vi "Crio9067_12chan.vi"() -> ()   [LabVIEW 2014]
uses:
  <vilib>/rvi/eio/nirviErrorMerge/nirviErrorMerge.xnode
  <vilib>/rvi/eio/common/nirviEmuClasses.ctl
  <vilib>/rvi/eio/common/nirviEmuTemplateMethod_errors.vi
  <vilib>/rvi/eio/nirviEIOMethodImplementation/nirviEIOMethodImplementation.xnode
  <vilib>/eio/EIOGrowableMethodNode/genericMethod/EIOGrowableMethodNode.xnode
  <vilib>/rvi/DataTransferAndStorage/Container/XNode/niFpgaContainer.xnode
  <vilib>/eio/EIONode/EIONode.xnode
  <vilib>/rvi/interface/RandomDataEmulation/nirviRandomDataFpgaReadWriteTemplate.vi
panel:
  in  "User Fpga Led":bool
  out "Chassis Temperature":i16
  in  "System Reset":bool
  in  "Sample Period (uSec)":u32=2
  out "Timed Out":bool
  out "Overwrite":bool
  out "Sample Gated":bool
  in  "USER FPGA LED":bool
  in  "Boolean":bool
  out "Stopped":bool
  out "nChannels":i32=8
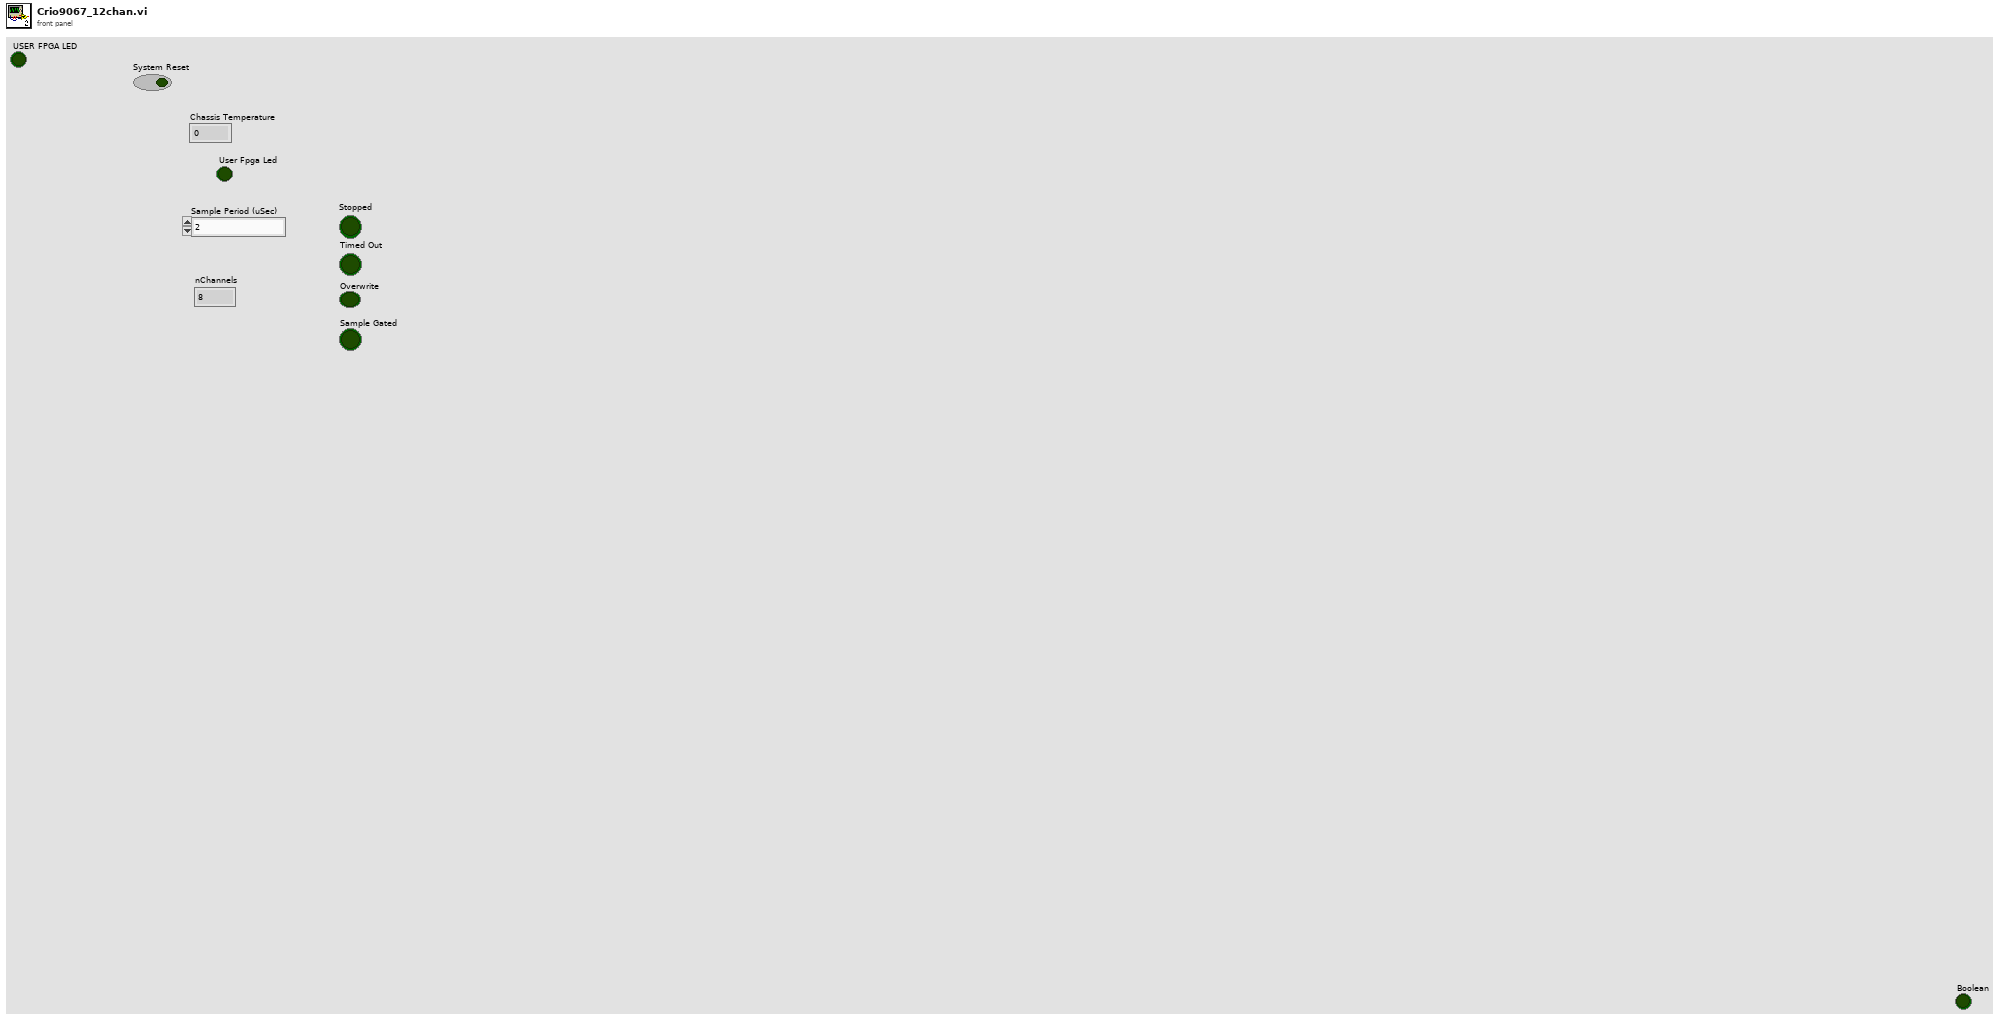
[diagram p1: front panel]
types:
  T1 = typedef "nirviEmuClasses.ctl" = enum16{"IO Read", "IO Write", "Method", "Property Read", "Property Write"}
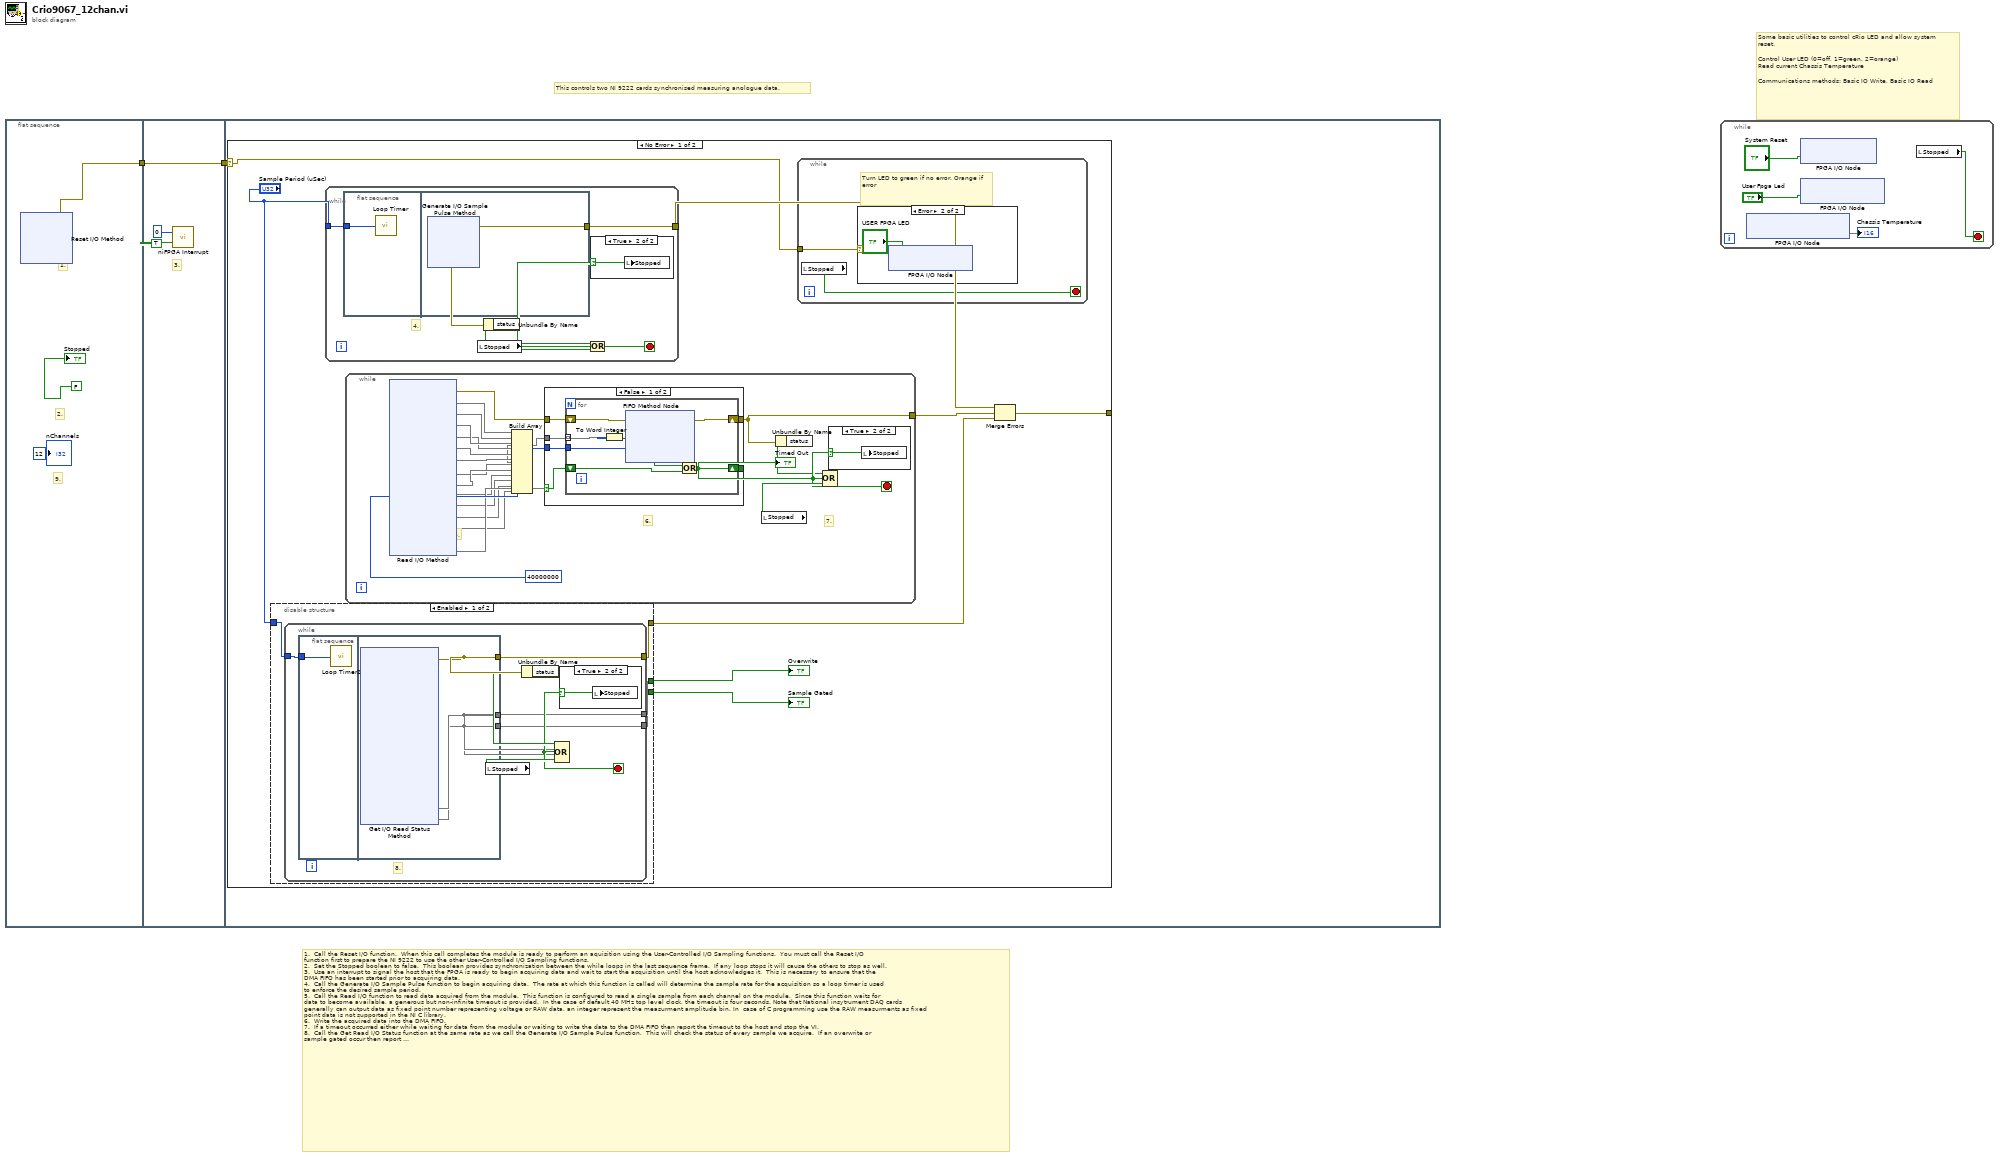
[diagram p0: block diagram]
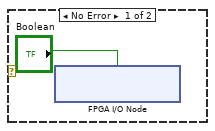
[diagram p2: hidden frame]
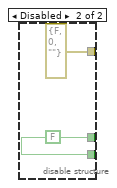
[diagram p4: hidden frame]
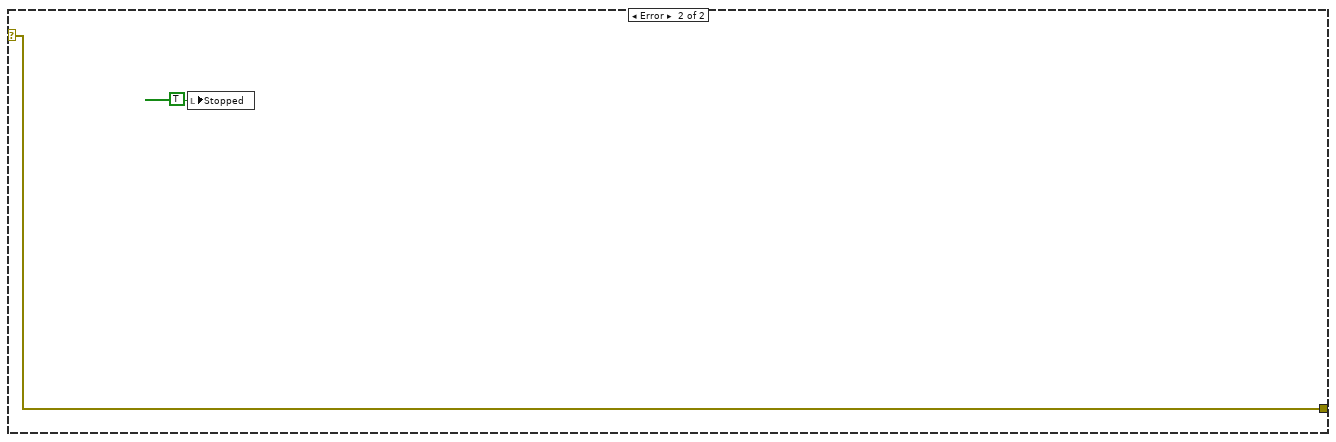
[diagram p8: hidden frame]
diagram:
  # "Some basic utilities to control cRio LED and allow system reset. \n\nControl User LED (0=off, 1=green, 2=orange)\nRead current Chassis Temperature\n\nCommunications methods: Basic IO Write, Basic IO Read"
  # "This controls two NI 9222 cards synchronised measuring anologue data."
  # "1.  Call the Reset I/O function.  When this call completes the module is ready to perform an aquisition using the User-Controlled I/O Sampling functions.  You must call the Reset I/O \nfunction first to prepare the NI 9222 to use the other User-Controlled I/O Sampling functions.\n2.  Set the Stopped boolean to false.  This boolean provides synchronization between the while loops in the last sequence frame.  If any loop stops it will cause the others to stop as well.\n3.  Use an interrupt to signal the host that the FPGA is ready to begin acquiring data and wait to start the acquisition until the host acknowledges it.  This is necessary to ensure that the \nDMA FIFO has been started prior to acquiring data.\n4.  Call the Generate I/O Sample Pulse function to begin acquiring data.  The rate at which this function is called will determine the sample rate for the acquisition so a loop timer is used\nto enforce the desired sample period.\n5.  Call the Read I/O function to read data acquired from the module.  This function is configured to read a single sample from each channel on the module.  Since this function waits for\ndata to become available, a generous but non-infinite timeout is provided.  In the case of default 40 MHz top level clock, the timeout is four seconds. Note that National insytrument DAQ cards \ngenerally can output data as fixed point number representing voltage or RAW data, an integer represent the measurment amplitude bin. In  case of C programming use the RAW measurments as fixed \npoint data is not supported in the NI C library. \n6.  Write the acquired data into the DMA FIFO.\n7.  If a timeout occurred either while waiting for data from the module or waiting to write the data to the DMA FIFO then report the timeout to the host and stop the VI.\n8.  Call the Get Read I/O Status function at the same rate as we call the Generate I/O Sample Pulse function.  This will check the status of every sample we acquire.  If an overwrite or \nsample gated occur then report the status to the host and stop the VI.  This loop is encased in a diagram disable struction to make it easily removable from the application.  Calling the \nGet Read I/O Status function is useful for development and debugging but not strictly necessary for deployment if there is no variable timing in the application.  In the above example, it\nis not possible to get a sample gated status unless the top loop's sample period is less than the minimum sample period supported by the module.  However, this application could \nproduce an overwrite status if the host VI cannot read from the DMA FIFO fast enough.\n9. I constant indicating the number of channels the FPGA is recording from. This is manually set."
  n1 = flat-sequence {
    tunnel: [w4] -> w2
    tunnel: w2 -> [w70]
    tunnel: [w70] -> w1
    tunnel: w1 -> [w73]
    frame #0 {
      # "9."
      # "2."
      # "1."
      n2 = xnode "Reset I/O Method"() -> ("error out"=w4:errorcluster)  [unwired: 1 in]
      "Stopped" <- FALSE ("Stopped")
      "nChannels" <- 12
    }
    frame #1 {
      # "3."
      n3 = call <vilib>:"niFPGA Interrupt.vi"("Wait Until Cleared (F)"=TRUE ("Wait Until Cleared"), "IRQ Number (0)"=u8 0 ("IRQ Number")) -> ()  [unwired: 1 in]
    }
    frame #2 {
      n4 = case shown="No Error" w73 {
        selector: w73 -> [w74 w1114]
        tunnel: [w78 w1114] -> _
        frame No Error {
          n5 = disable-structure shown="Enabled" {
            disable-tunnel: [w89 errorcluster {"status"=FALSE, "code"=0, "source"=""} ("error out")] -> w79
            disable-tunnel: "Sample Period (uSec)" -> [w88 _]
            disable-tunnel: [w87 w534] -> w75
            disable-tunnel: [w86 w534] -> w76
            frame Enabled {
              n6 = while {
                tunnel: [w96] -> w89
                tunnel: w88 -> [w95]
                tunnel: [w91] -> w87
                tunnel: [w90] -> w86
                stop <- w92 stop-if-true
                # "8."
                n7 = flat-sequence {
                  tunnel: w95 -> [w98]
                  tunnel: [w101] -> w96
                  tunnel: [w100] -> w91
                  tunnel: [w99] -> w90
                  frame #0 {
                    n8 = call "Loop Timer2"("Count(uSec)"=w98) -> ()  [unwired: 1 out]
                  }
                  frame #1 {
                    n9 = xnode "Get I/O Read Status Method"() -> ("error out"=w101:errorcluster, "Overwrite"=w100, "Sample Gated"=w99)  [unwired: 1 in]
                  }
                }
                n10 = local read "Stopped"() -> (w94:bool)
                n11 = Unbundle By Name(w96) -> ("status"=w93:bool)
                n12 = Compound Arithmetic op=OR(w93, w91, w90, w94) -> (w92:bool)
                n13 = case shown="True" w92 {
                  selector: w92 -> [_ w97]
                  frame False {
                  }
                  frame True {
                    n14 = local write "Stopped"(w97) -> ()
                  }
                }
              }
            }
            frame Disabled {
              w534 = FALSE ("Overwrite")
            }
          }
          "Overwrite" <- w75
          "Sample Gated" <- w76
          n15 = while {
            tunnel: "Sample Period (uSec)" -> [w1046]
            tunnel: [w1043] -> w81
            stop <- w1042 stop-if-true
            # "4."
            n16 = flat-sequence {
              tunnel: w1046 -> [w1048]
              tunnel: [w1049] -> w1043
              frame #0 {
                n17 = call "Loop Timer"("Count(uSec)"=w1048) -> ()  [unwired: 1 out]
              }
              frame #1 {
                n18 = xnode "Generate I/O Sample Pulse Method"() -> ("error out"=w1049:errorcluster)  [unwired: 1 in]
              }
            }
            n19 = local read "Stopped"() -> (w1045:bool)
            n20 = Unbundle By Name(w1043) -> ("status"=w1044:bool)
            n21 = Or(x=w1044, y=w1045) -> (x .or. y?=w1042:bool)
            n22 = case shown="True" w1042 {
              selector: w1042 -> [_ w1047]
              frame False {
              }
              frame True {
                n23 = local write "Stopped"(w1047) -> ()
              }
            }
          }
          n24 = while {
            tunnel: [w554] -> w80
            stop <- w541 stop-if-true
            w555 = 40000000 ("Timeout")
            # "7."
            # "6."
            # "5."
            n25 = xnode "Read I/O Method"("Timeout"=w555) -> ("error out"=w553:errorcluster, "Mod1/AI0"=w543, "Mod1/AI1"=w556, "Mod1/AI2"=w549, "Mod1/AI3"=w548, "Mod2/AI0"=w547, "Mod2/AI1"=w546, "Mod2/AI2"=w544, "Mod2/AI3"=w545, "Mod3/AI0"=w539, "Mod3/AI1"=w538, "Mod3/AI2"=w537, "Mod3/AI3"=w536, "Timed Out"=w552)  [unwired: 1 in]
            n26 = Build Array(w543, w556, w549, w548, w547, w546, w544, w545, w539, w538, w537, w536) -> (w542:void[])
            n27 = case shown="False" w552 {
              selector: w552 -> [w559 w572]
              tunnel: w555 -> [w563 _]
              tunnel: [w562 w573] -> w554
              tunnel: [w561 w572] -> w550
              tunnel: w553 -> [w560 w573]
              tunnel: w542 -> [w558 _]
              frame False {
                n28 = for {
                  tunnel: w558 -> [w564] mode=indexing
                  shift-right: [w570] -> w562
                  shift-left: w560 -> [w571]
                  tunnel: w563 -> [w569]
                  shift-right: [w567] -> w561
                  shift-left: w559 -> [w566]
                  n29 = To Word Integer(number=w564) -> (16bit integer=w565:i16)
                  n30 = xnode ("FIFO Method Node")("Element"=w565, "Timeout"=w569, "error in (no error)"=w571) -> ("Timed Out?"=w568:bool, "error out"=w570:errorcluster)  [unwired: 1 in, 1 out]
                  n31 = Or(x=w568, y=w566) -> (x .or. y?=w567:bool)
                }
              }
              frame True {
              }
            }
            "Timed Out" <- w550
            n32 = local read "Stopped"() -> (w551:bool)
            n33 = Unbundle By Name(w554) -> ("status"=w540:bool)
            n34 = Compound Arithmetic op=OR(w540, w550, w551) -> (w541:bool)
            n35 = case shown="True" w541 {
              selector: w541 -> [_ w557]
              frame False {
              }
              frame True {
                n36 = local write "Stopped"(w557) -> ()
              }
            }
          }
          n37 = while {
            tunnel: w74 -> [w83]
            stop <- w82 stop-if-true
            # "Turn LED to green if no error. Orange if error"
            n38 = local read "Stopped"() -> (w82:bool)
            n39 = case shown="Error" w83 {
              frame No Error {
                n40 = xnode "FPGA I/O Node"("USER FPGA LED"="Boolean") -> ()  [unwired: 1 in, 1 out]
              }
              frame Error {
                n41 = xnode "FPGA I/O Node"("USER FPGA LED"="USER FPGA LED") -> ()  [unwired: 1 in, 1 out]
              }
            }
          }
          n42 = Merge Errors(w81, w80, w79) -> (w78:errorcluster)
        }
        frame Error {
          n43 = local write "Stopped"(TRUE ("Stopped")) -> ()
        }
      }
    }
  }
  n44 = while {
    stop <- w1116 stop-if-true
    n45 = xnode "FPGA I/O Node"() -> ("Chassis Temperature"=→"Chassis Temperature")  [unwired: 1 in, 1 out]
    n46 = xnode "FPGA I/O Node"("System Reset"="System Reset") -> ()  [unwired: 1 in, 1 out]
    n47 = xnode "FPGA I/O Node"("USER FPGA LED"="User Fpga Led") -> ()  [unwired: 1 in, 1 out]
    n48 = local read "Stopped"() -> (w1116:bool)
  }
